vi "nirviWait.vi"(1 "Count(Ticks)":u32) -> (0 "Tick Count(Ticks)":u32)   [LabVIEW 2017]
doc: "Delays for a certain time interval before the output data dependence becomes valid."
panel:
  in  "Counter Units":u16(ring) items=["Ticks", "uSec", "mSec"]
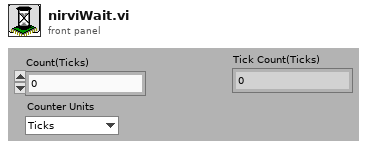
[diagram p1: front panel]
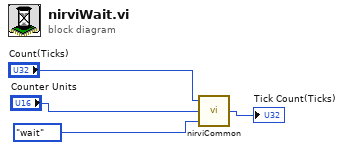
[diagram p0: block diagram]
diagram:
  n1 = call <vilib>:"nirviCommon.vi"("Action"=enum16{"wait", "wait multiple", "tick count"}."wait", "Counter Units"="Counter Units", "Count(uSec)"="Count(Ticks)") -> ("Tick Count(uSec)"=→"Tick Count(Ticks)":u32)
